vi "Read SubObj.vi"(8 "error in (no error)":errorcluster, 11 "ShortcutMenuActivationMsg in":refnum<class "ShortcutMenuActivationMsg.lvclass">) -> (0 "error out":errorcluster, 2 "SubObj":refnum<vi>, 3 "ShortcutMenuActivationMsg out":refnum<class "ShortcutMenuActivationMsg.lvclass">)   [LabVIEW 2015, in "ActorEvents.lvlib" / "ShortcutMenuActivationMsg.lvclass"]
uses:
  ShortcutMenuActivationMsg.lvclass
  ShortcutMenuActivationMsg.lvclass/ShortcutMenuActivationMsg.ctl
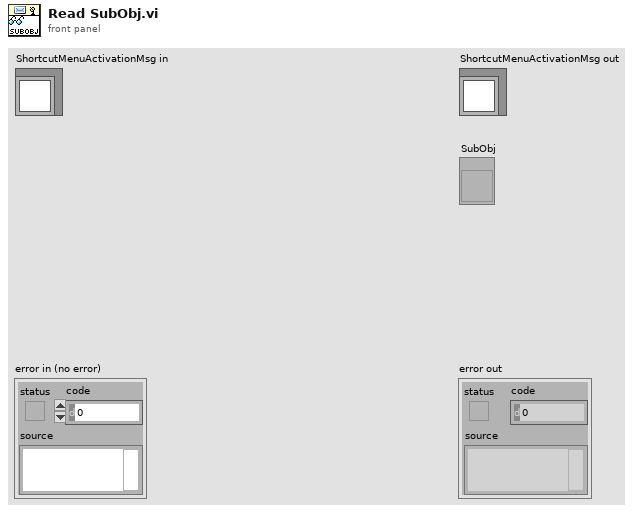
[diagram p1: front panel]
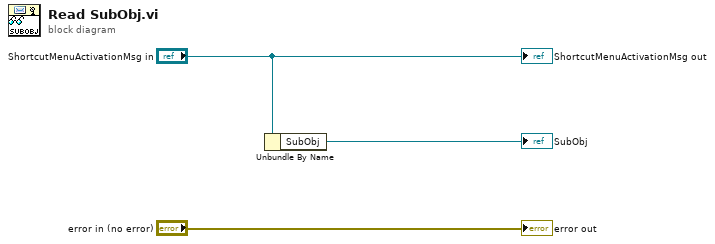
[diagram p0: block diagram]
diagram:
  n1 = Unbundle By Name("ShortcutMenuActivationMsg in") -> ("SubObj"=→"SubObj":refnum<vi>)
  "error out" <- "error in (no error)"
  "ShortcutMenuActivationMsg out" <- "ShortcutMenuActivationMsg in"
